vi "string concatinate.vi"() -> ()   [LabVIEW 2020]
panel:
  in  "Urban/ Rural":string
  in  "track no.":string
  in  "batch":string
  out "output":string
  in  "School":string
  in  "Name":string
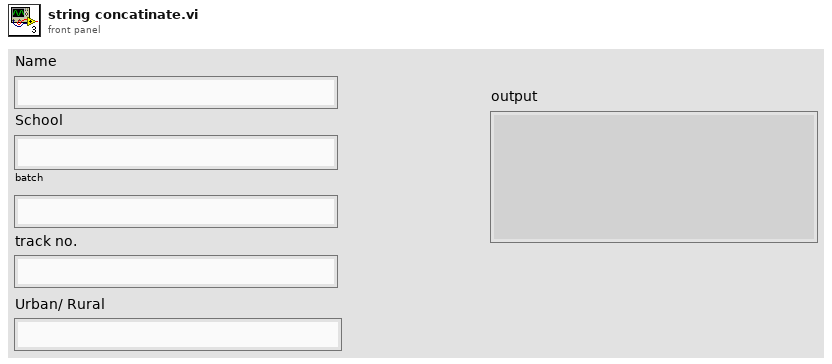
[diagram p1: front panel]
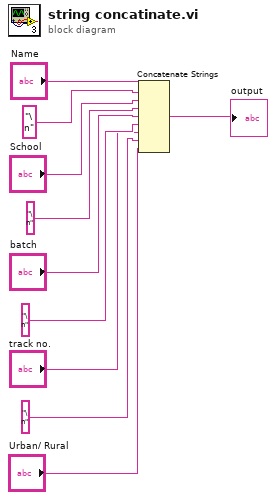
[diagram p0: block diagram]
diagram:
  n1 = Concatenate Strings("Name", "\n" ("string"), "School", "\n" ("string"), "batch", "\n", "track no.", "\n", "Urban/ Rural") -> (→"output":string)
